vi "Current_Filepath.vi"(2 "Short_Name":string, 3 "Filename in":path, 4 "Data Type":string="Calibrations") -> (0 "Filename Out":path, 1 "Directory":path)   [LabVIEW 2015]
uses:
  Globals/Meas_global.vi
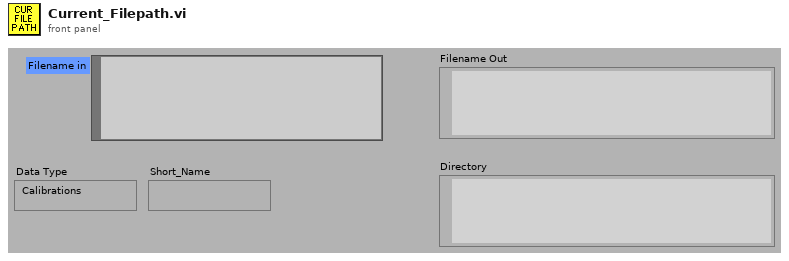
[diagram p1: front panel]
types:
  T1 = typedef "Post_Process.ctl" = enum16{"Take New Data", "Post Process Raw Data File"}
  T2 = typedef "LVDateTimeRec.ctl" = cluster{"fractional second":dbl, "second":i32, "minute":i32, "hour":i32, "day of month":i32, "month":i32, "year":i32, "day of week":i32, "day of year":i32, "DST":i32}
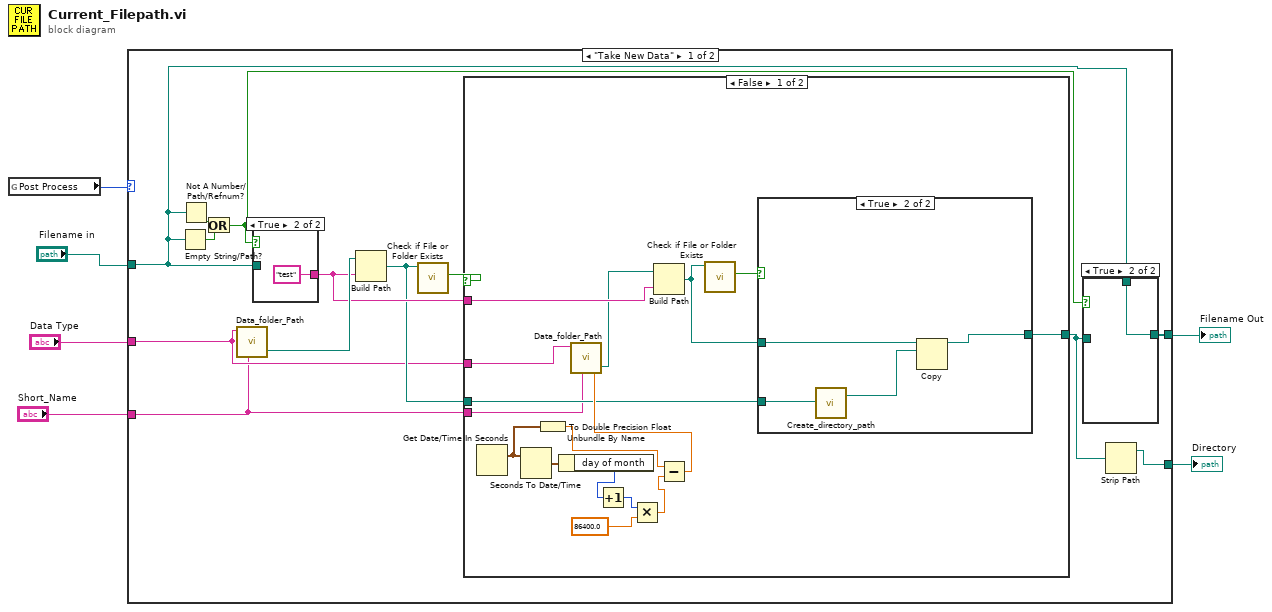
[diagram p0: block diagram]
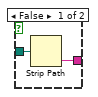
[diagram p3: hidden frame]
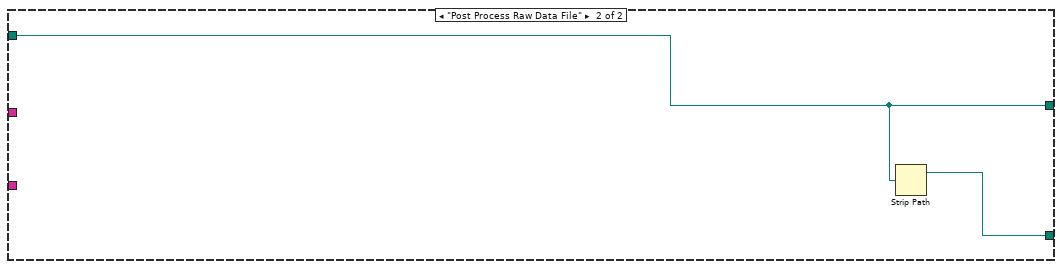
[diagram p6: hidden frame]
diagram:
  n1 = global read "Meas_global.vi" "Post Process"() -> (w3:T1)
  n2 = case shown="\"Take New Data\"" w3 {
    tunnel: "Filename in" -> [w8 w48]
    tunnel: "Data Type" -> [w15 _]
    tunnel: [w11 w48] -> w4
    tunnel: [w9 w47] -> w2
    tunnel: "Short_Name" -> [w7 _]
    frame "Take New Data" {
      n3 = Empty String/Path?(string/path=w8) -> (empty?=w13:bool)
      n4 = Not A Number/Path/Refnum?(number/path/refnum=w8) -> (NaN/Path/Refnum?=w14:bool)
      n5 = Or(x=w14, y=w13) -> (x .or. y?=w12:bool)
      n6 = call "Data_folder_Path.vi"("Data Type"=w15, "Short_Name"=w7) -> ("Data Folder"=w19:path)  [unwired: 4 in]
      n7 = case shown="True" w12 {
        tunnel: [w23 "test" ("name")] -> w17
        tunnel: w8 -> [w22 _]
        frame False {
          n8 = Strip Path(path=w22) -> (name=w23:string)  [unwired: 1 out]
        }
        frame True {
        }
      }
      n9 = Build Path(base path=w19, name or relative path=w17) -> (appended path=w16:path)
      n10 = call <vilib>:"Check if File or Folder Exists.vi"("path"=w16) -> ("file or folder exists?"=w18:bool)  [unwired: 1 in, 9 out]
      n11 = case shown="False" w18 {
        tunnel: w15 -> [w34 _]
        tunnel: w17 -> [w39 _]
        tunnel: w16 -> [w37 w46]
        tunnel: [w35 w46] -> w10
        tunnel: w7 -> [w25 _]
        frame False {
          n12 = Get Date/Time In Seconds() -> (seconds since 1Jan1904=w28:timestamp)
          n13 = Seconds To Date/Time(time stamp (now)=w28) -> (date time rec=w33:T2)  [unwired: 1 in]
          n14 = To Double Precision Float(number=w28) -> (double precision float=w27:dbl)
          n15 = Unbundle By Name(w33) -> ("day of month"=w32:i32)
          n16 = Increment(x=w32) -> (x+1=w31:i32)
          n17 = Multiply(x=w31, y=86400.0) -> (x*y=w29:dbl)
          n18 = Subtract(x=w27, y=w29) -> (x-y=w40:dbl)
          n19 = call "Data_folder_Path.vi"("Data Type"=w34, "Short_Name"=w25, "seconds"=w40) -> ("Data Folder"=w26:path)  [unwired: 3 in]
          n20 = Build Path(base path=w26, name or relative path=w39) -> (appended path=w36:path)
          n21 = call <vilib>:"Check if File or Folder Exists.vi"("path"=w36) -> ("file or folder exists?"=w38:bool)  [unwired: 1 in, 9 out]
          n22 = case shown="True" w38 {
            tunnel: w36 -> [_ w45]
            tunnel: w37 -> [w41 w43]
            tunnel: [w41 w44] -> w35
            frame False {
            }
            frame True {
              n23 = call "Create_directory_path.vi"("Path name"=w43) -> ("Path name Out"=w42:path)  [unwired: 2 in, 1 out]
              n24 = Copy(10:w42, 11:w45) -> (3:w44:path)  [unwired: 3 in, 2 out]
            }
          }
        }
        frame True {
        }
      }
      n25 = case shown="True" w12 {
        tunnel: w10 -> [w20 _]
        tunnel: [w20 w21] -> w11
        tunnel: w8 -> [_ w21]
        frame False {
        }
        frame True {
        }
      }
      n26 = Strip Path(path=w10) -> (stripped path=w9:path)  [unwired: 1 out]
    }
    frame "Post Process Raw Data File" {
      n27 = Strip Path(path=w48) -> (stripped path=w47:path)  [unwired: 1 out]
    }
  }
  "Filename Out" <- w4
  "Directory" <- w2
